vi "Wait for Response Message.vi"(8 "error in (no error)":errorcluster, 9 "timeout in ms":i32, 11 "Process In":refnum<class "Debug Process.lvclass">) -> (0 "error out":errorcluster, 1 "Message Data":variant, 2 "Message":string, 3 "Process Out":refnum<class "Debug Process.lvclass">, 4 "timed out?":bool)   [LabVIEW 2020, in "Debug Process.lvclass"]
uses:
  Debug Process.lvclass
  Debug Process.lvclass/Debug Process.ctl
  <vilib>/Utility/error.llb/Error Cluster From Error Code.vi
  <vilib>/ErrorRing/Error Ring.xnode
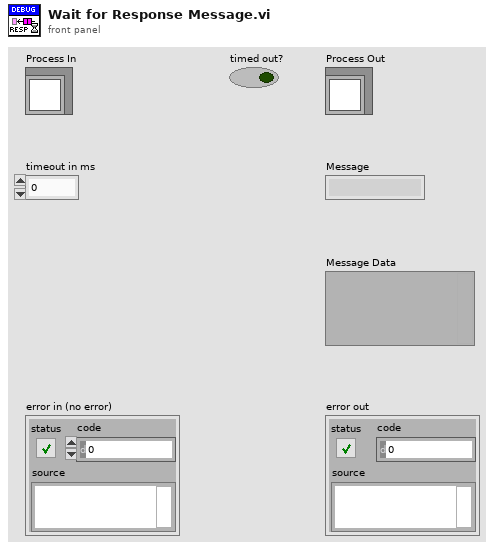
[diagram p1: front panel]
types:
  T1 = typedef "Debug Process.lvclass/Lifecycle State.ctl" = enum16{"Uninitialized", "Initialized", "Started", "Running", "Stopped", "Finished"}
  T2 = typedef "Debug Process.lvclass/Request Message Cluster.ctl" = cluster{"Message":string, "Message Data":variant, "Request Error":errorcluster}
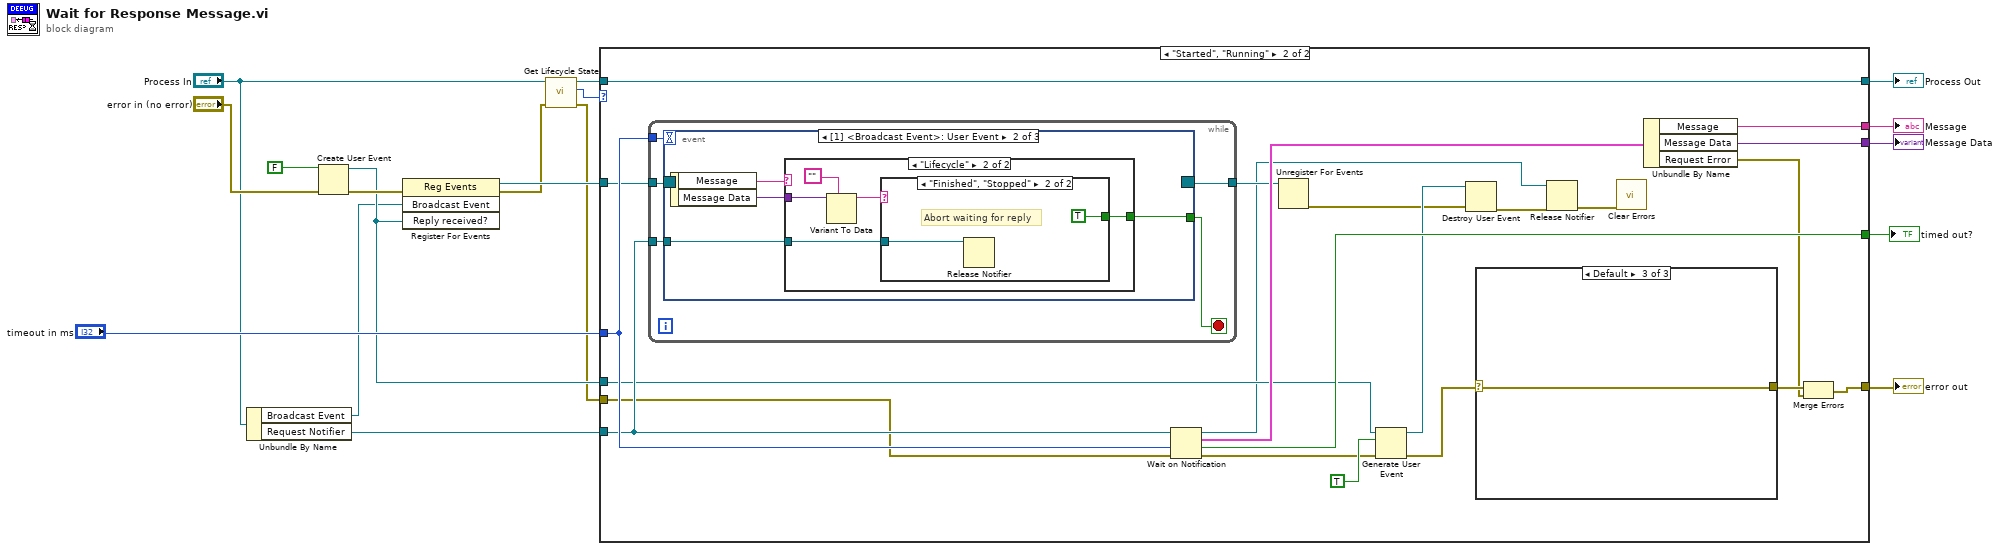
[diagram p0: block diagram]
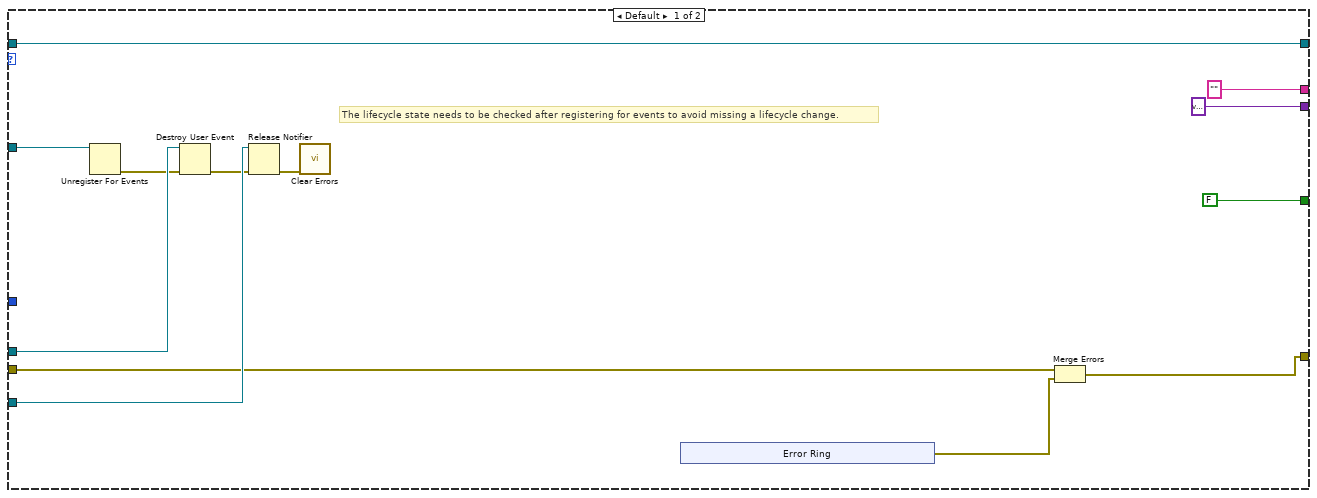
[diagram p2: hidden frame]
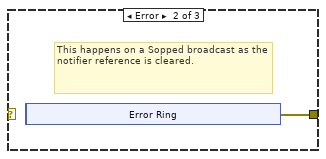
[diagram p4: hidden frame]
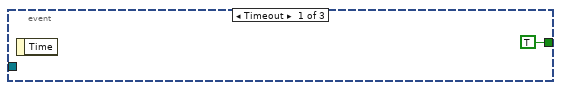
[diagram p5: hidden frame]
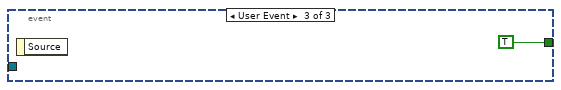
[diagram p8: hidden frame]
diagram:
  n1 = Unbundle By Name("Process In") -> ("Broadcast Event"=w6:refnum<user-event>, "Request Notifier"=w9:refnum<notifier>)
  n2 = Create User Event(user event datatype=FALSE ("Reply received?"), error in="error in (no error)") -> (user event=w7:refnum<user-event>, error out=w17:errorcluster)
  n3 = register-events(error in=w17, w6, w7) -> (reference out=w14:refnum<event-registration>, error out=w5:errorcluster)  [unwired: 1 in]
  n4 = call "Get Lifecycle State.vi"("error in (no error)"=w5, "Process In"="Process In") -> ("error out"=w4:errorcluster, "Lifecycle State"=w1:T1, "Process Out"=w2:refnum<class "Debug Process.lvclass">)  [unwired: 6 in, 1 out]
  n5 = case shown="\"Started\", \"Running\"" w1 {
    tunnel: "timeout in ms" -> [_ w57]
    tunnel: w14 -> [w25 w56]
    tunnel: [variant ("Message Data") w55] -> w13
    tunnel: ["" ("Message") w54] -> w12
    tunnel: [FALSE ("timed out?") w52] -> w11
    tunnel: w9 -> [w23 w51]
    tunnel: [w30 w37] -> w8
    tunnel: w7 -> [w24 w47]
    tunnel: w4 -> [w20 w39]
    tunnel: [w31 w38] -> w3
    tunnel: w2 -> [w31 w38]
    frame Default {
      # "The lifecycle state needs to be checked after registering for events to avoid missing a lifecycle change."
      n6 = Unregister For Events(event registration refnum=w25) -> (error out=w22:errorcluster)  [unwired: 1 in]
      n7 = Destroy User Event(user event=w24, error in=w22) -> (error out=w21:errorcluster)
      n8 = Release Notifier(notifier=w23, error in (no error)=w21) -> (error out=w19:errorcluster)  [unwired: 1 in, 2 out]
      n9 = call <vilib>:"Clear Errors.vi"("error in (no error)"=w19) -> ()  [unwired: 5 in, 2 out]
      n10 = xnode "Error Ring"() -> ("error out"=w29:errorcluster)
      n11 = Merge Errors(w20, w29) -> (w30:errorcluster)
    }
    frame "Started", "Running" {
      n12 = while {
        tunnel: w56 -> [w73]
        tunnel: w57 -> [w72]
        tunnel: w51 -> [w70]
        tunnel: [w69] -> w50
        stop <- w71 stop-if-true
        n13 = event shown="[1] <Broadcast Event>: User Event" {
          selector: w73 -> [_ _ _]
          dyn-events: [_ _ _] -> w69
          timeout: w72 -> [_ _ _]
          tunnel: [TRUE w75 TRUE] -> w71
          tunnel: w70 -> [_ w76 _]
          event Timeout {
            n14 = event-data() -> ()  [unwired: 1 in, 1 out]
          }
          event User Event {
            n15 = event-data() -> ("Message"=w78:string, "Message Data"=w77:variant)  [unwired: 1 in]
            n16 = case shown="\"Lifecycle\"" w78 {
              tunnel: w77 -> [_ w83]
              tunnel: w76 -> [_ w80]
              tunnel: [_ w79] -> w75
              frame Default {
              }
              frame "Lifecycle" {
                n17 = Variant To Data(type="", Variant=w83) -> (data=w81:string)  [unwired: 1 in, 1 out]
                n18 = case shown="\"Finished\", \"Stopped\"" w81 {
                  tunnel: w80 -> [_ w85]
                  tunnel: [_ TRUE] -> w79
                  frame Default {
                  }
                  frame "Finished", "Stopped" {
                    # "Abort waiting for reply"
                    n19 = Release Notifier(notifier=w85) -> ()  [unwired: 2 in, 3 out]
                  }
                }
              }
            }
          }
          event User Event {
            n20 = event-data() -> ()  [unwired: 1 in, 1 out]
          }
        }
      }
      n21 = Wait on Notification(notifier=w51, timeout in ms (-1)=w57, error in (no error)=w39) -> (notifier out=w41:refnum<notifier>, notification=w53:T2, timed out?=w52:bool, error out=w43:errorcluster)  [unwired: 1 in]
      n22 = Unregister For Events(event registration refnum=w50) -> (error out=w45:errorcluster)  [unwired: 1 in]
      n23 = Generate User Event(user event=w47, event data cluster=TRUE ("event data"), error in=w43) -> (user event out=w46:refnum<user-event>, error out=w48:errorcluster)  [unwired: 1 in]
      n24 = Destroy User Event(user event=w46, error in=w45) -> (error out=w42:errorcluster)
      n25 = case shown="Default" w48 {
        selector: w48 -> [w58 _ w68]
        tunnel: [w58 w59 w68] -> w49
        frame No Error {
        }
        frame Error {
          # "This happens on a Sopped broadcast as the notifier reference is cleared."
          n26 = xnode "Error Ring"() -> ()  [unwired: 1 out]
          n27 = xnode "Error Ring"() -> ("error out"=w59:errorcluster)
        }
        frame Default {
        }
      }
      n28 = Release Notifier(notifier=w41, error in (no error)=w42) -> (error out=w40:errorcluster)  [unwired: 1 in, 2 out]
      n29 = call <vilib>:"Clear Errors.vi"("error in (no error)"=w40) -> ()  [unwired: 5 in, 2 out]
      n30 = Unbundle By Name(w53) -> ("Message"=w54:string, "Message Data"=w55:variant, "Request Error"=w36:errorcluster)
      n31 = Merge Errors(w49, w36) -> (w37:errorcluster)
    }
  }
  "Process Out" <- w3
  "error out" <- w8
  "Message Data" <- w13
  "Message" <- w12
  "timed out?" <- w11
